vi "Swerve Drive.vi"(0 "X":dbl(slide) scale=-1.0..1.0, 1 "Rot. Point Y":dbl, 3 "Rot. Point X":dbl, 4 "Back Left":bool, 6 "Back Right":bool, 7 "Y":dbl(slide) scale=1.0..-1.0, 8 "Front Left":bool, 10 "Front Right":bool, 11 "Z":dbl(knob) scale=1.0..-1.0, 12 "Auto Controls":bool, 13 "Robot-Centric":bool) -> (15 "Debug is on":bool)   [LabVIEW 2016, in "CAN Talon SRX Swerve.lvlib"]
uses:
  CAN Talon SRX Swerve.lvlib
  <vilib>/Rock Robotics/WPI/ThirdParty/CanMotor/TalonSRX/WPI_CANTalonSRX_APIControlMode.ctl
  Apple Gyro/Apple Pi Gyro Library.lvlib
panel:
  in  "Deadband":dbl=0.04 format="%#_13g"
  in  "Robot Length":dbl=21.5
  in  "Robot Width":dbl=29.5
  # "SWERVE DRIVE\nVersion 3.2\n\nCory Lynch\nChris Garuti\nApple Pi Robotics\nTeam 2067"
  # "Debug"
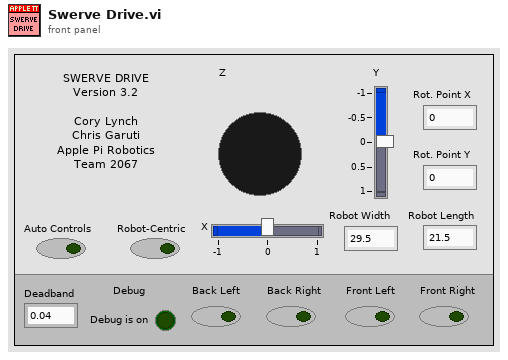
[diagram p1: front panel]
types:
  T1 = typedef "WPI_CANTalonSRX_APIControlMode.ctl" = enum8{"Percent VBus", "Speed", "Position", "Slave", "Unchanged / Invalid", "Voltage Compensation", "Current", "Motion Profile", "Motion Magic"}
  T2 = enum16{"Back Left", "Back Right", "Front Left", "Front Right"}
  T3 = typedef "WPI_MotorControlDeviceRef.ctl" = cluster{"DeviceStatus":errorcluster, "Type":T4, "PWM":cluster{"PWM Channel":T5, "DeadBand":T6}, "CAN":cluster{"Device Number":u8, "SetOutput VI Ref":variant, "GetOutput VI Ref":variant, "Enable VI Ref":variant, "Disable VI Ref":variant, "Data":variant}, "Invert":bool}
  T4 = typedef "WPI_MotorControlType.ctl" = enum16{"PWM", "CAN"}
  T5 = typedef "FPGA_DIOPWMChannel.ctl" = enum8{"PWM 0", "PWM 1", "PWM 2", "PWM 3", "PWM 4", "PWM 5", "PWM 6", "PWM 7", "PWM 8", "PWM 9", "PWM MXP 0", "PWM MXP 1", "PWM MXP 2", "PWM MXP 3", "PWM MXP 4", "PWM MXP 5", "PWM MXP 6", "PWM MXP 7", "PWM MXP 8", "PWM MXP 9", "Invalid"}
  T6 = typedef "WPI_PWMDeadband.ctl" = cluster{"Name":string, "maxPositivePwm":i32, "minPositivePwm":i32, "centerPwm":i32, "maxNegativePwm":i32, "minNegativePwm":i32, "angularRange":u16}
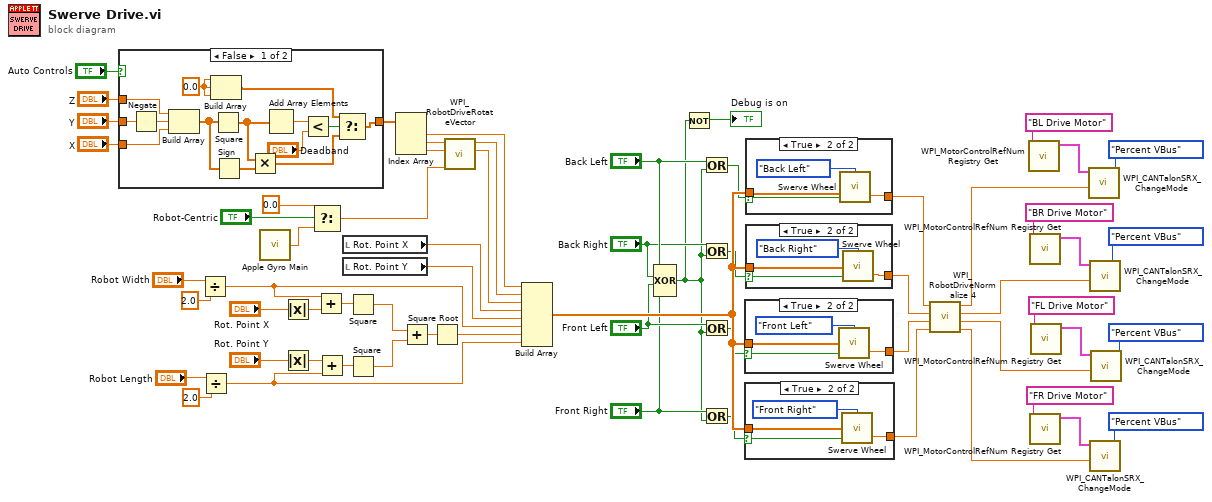
[diagram p0: block diagram]
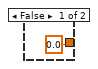
[diagram p2: hidden frame]
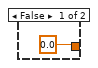
[diagram p3: hidden frame]
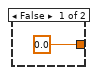
[diagram p4: hidden frame]
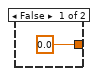
[diagram p5: hidden frame]
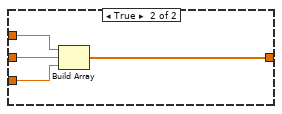
[diagram p6: hidden frame]
diagram:
  n1 = case shown="False" "Auto Controls" {
    tunnel: "Y" -> [w74 w80]
    tunnel: "X" -> [w68 w81]
    tunnel: "Z" -> [w64 w78]
    tunnel: [w65 w79] -> w24
    frame False {
      w72 = 0.0 ("element")
      n2 = Negate(x=w74) -> (-x=w67:dbl)
      n3 = Build Array(w64, w67, w68) -> (w71:dbl[])
      n4 = Build Array(w72, w72, w72) -> (w73:dbl[])
      n5 = Square(x=w71) -> (x^2=w69:dbl[])
      n6 = Sign(1:w71) -> (0:w70:dbl[])
      n7 = Multiply(x=w69, y=w70) -> (x*y=w66:dbl[])
      n8 = Add Array Elements(numeric array=w69) -> (sum=w77:dbl)
      n9 = Less?(x=w77, y="Deadband") -> (x < y?=w75:bool)
      n10 = Select(t=w73, s=w75, f=w66) -> (s? t:f=w65:dbl[])
    }
    frame True {
      n11 = Build Array(w78, w80, w81) -> (w79:dbl[])
    }
  }
  n12 = Divide(x="Robot Width", y=2.0) -> (x/y=w28:dbl)
  n13 = Divide(x="Robot Length", y=2.0) -> (x/y=w26:dbl)
  n14 = call "Apple Gyro Main.vi"() -> ("Gyro Yaw Out"=w15:dbl)  [unwired: 4 in]
  n15 = Absolute Value(x="Rot. Point X") -> (abs(x)=w46:dbl)
  n16 = Absolute Value(x="Rot. Point Y") -> (abs(x)=w44:dbl)
  n17 = Select(t=0.0, s="Robot-Centric", f=w15) -> (s? t:f=w19:dbl)
  n18 = Add(x=w28, y=w46) -> (x+y=w45:dbl)
  n19 = Add(x=w44, y=w26) -> (x+y=w43:dbl)
  n20 = local read "Rot. Point X"() -> (w30:dbl)
  n21 = local read "Rot. Point Y"() -> (w29:dbl)
  n22 = Square(x=w45) -> (x^2=w41:dbl)
  n23 = Square(x=w43) -> (x^2=w42:dbl)
  n24 = Index Array(array=w24) -> (element #1=w18:dbl, element #2=w25:dbl, element #3=w33:dbl)  [unwired: 3 in]
  n25 = Add(x=w41, y=w42) -> (x+y=w40:dbl)
  n26 = Square Root(x=w40) -> (sqrt(x)=w27:dbl)
  n27 = call <vilib>:"WPI_RobotDriveRotateVector.vi"("Angle"=w19, "X"=w33, "Y"=w25) -> ("X'"=w22:dbl, "Y'"=w17:dbl)  [unwired: 7 out]
  n28 = Build Array(w18, w17, w22, w30, w29, w28, w27, w26) -> (w23:dbl[])
  n29 = Compound Arithmetic op=XOR("Back Left", "Back Right", "Front Left", "Front Right") -> (w6:bool)
  n30 = Not(x=w6) -> (.not. x?=→"Debug is on":bool)
  n31 = Or(x="Back Left", y=w6) -> (x .or. y?=w14:bool)
  n32 = Or(x="Back Right", y=w6) -> (x .or. y?=w13:bool)
  n33 = Or(x="Front Left", y=w6) -> (x .or. y?=w12:bool)
  n34 = Or(x="Front Right", y=w6) -> (x .or. y?=w11:bool)
  n35 = case shown="True" w12 {
    selector: w12 -> [_ w83]
    tunnel: [0.0 ("Speed") w85] -> w61
    tunnel: w23 -> [_ w84]
    frame False {
    }
    frame True {
      n36 = call "Swerve Wheel.vi"("Wheel"=T2."Front Left", "Debug?"=w83, "Inputs"=w84) -> ("Speed"=w85:dbl)  [unwired: 2 in]
    }
  }
  n37 = case shown="True" w11 {
    selector: w11 -> [_ w88]
    tunnel: [0.0 ("Speed") w90] -> w60
    tunnel: w23 -> [_ w89]
    frame False {
    }
    frame True {
      n38 = call "Swerve Wheel.vi"("Wheel"=T2."Front Right", "Debug?"=w88, "Inputs"=w89) -> ("Speed"=w90:dbl)  [unwired: 2 in]
    }
  }
  n39 = case shown="True" w14 {
    selector: w14 -> [_ w93]
    tunnel: [0.0 ("Speed") w96] -> w63
    tunnel: w23 -> [_ w94]
    frame False {
    }
    frame True {
      n40 = call "Swerve Wheel.vi"("Wheel"=T2."Back Left", "Debug?"=w93, "Inputs"=w94) -> ("Speed"=w96:dbl)  [unwired: 2 in]
    }
  }
  n41 = case shown="True" w13 {
    selector: w13 -> [_ w98]
    tunnel: [0.0 ("Speed") w100] -> w62
    tunnel: w23 -> [_ w99]
    frame False {
    }
    frame True {
      n42 = call "Swerve Wheel.vi"("Wheel"=T2."Back Right", "Debug?"=w98, "Inputs"=w99) -> ("Speed"=w100:dbl)  [unwired: 2 in]
    }
  }
  n43 = call <vilib>:"WPI_RobotDriveNormalize 4.vi"("D"=w60, "C"=w61, "B"=w62, "A"=w63) -> ("D'"=w48:dbl, "C'"=w49:dbl, "B'"=w50:dbl, "A'"=w51:dbl)
  n44 = call <vilib>:"WPI_MotorControlRefNum Registry Get.vi"("refnum name"="BL Drive Motor") -> ("MotorControlDevRef"=w59:T3)  [unwired: 9 in, 1 out]
  n45 = call <vilib>:"WPI_MotorControlRefNum Registry Get.vi"("refnum name"="BR Drive Motor") -> ("MotorControlDevRef"=w56:T3)  [unwired: 9 in, 1 out]
  n46 = call <vilib>:"WPI_MotorControlRefNum Registry Get.vi"("refnum name"="FR Drive Motor") -> ("MotorControlDevRef"=w52:T3)  [unwired: 9 in, 1 out]
  n47 = call <vilib>:"WPI_MotorControlRefNum Registry Get.vi"("refnum name"="FL Drive Motor") -> ("MotorControlDevRef"=w55:T3)  [unwired: 9 in, 1 out]
  n48 = call <vilib>:"WPI_CANTalonSRX_ChangeMode.vi"("Output"=w51, "Control Mode"=WPI_CANTalonSRX_APIControlMode."Percent VBus", "CAN Talon SRX Ref"=w59) -> ()  [unwired: 7 in, 2 out]
  n49 = call <vilib>:"WPI_CANTalonSRX_ChangeMode.vi"("Output"=w50, "Control Mode"=WPI_CANTalonSRX_APIControlMode."Percent VBus", "CAN Talon SRX Ref"=w56) -> ()  [unwired: 7 in, 2 out]
  n50 = call <vilib>:"WPI_CANTalonSRX_ChangeMode.vi"("Output"=w48, "Control Mode"=WPI_CANTalonSRX_APIControlMode."Percent VBus", "CAN Talon SRX Ref"=w52) -> ()  [unwired: 7 in, 2 out]
  n51 = call <vilib>:"WPI_CANTalonSRX_ChangeMode.vi"("Output"=w49, "Control Mode"=WPI_CANTalonSRX_APIControlMode."Percent VBus", "CAN Talon SRX Ref"=w55) -> ()  [unwired: 7 in, 2 out]
